vi "Ka2tesla - Hybrid.vi"(1 "SC Current [kA]":dbl format="%.5f", 2 "Current [KA]":dbl format="%.5f") -> (0 "Field":dbl=1.0 format="%.4f")   [LabVIEW 2020]
uses:
  PS Comm Globals.vi
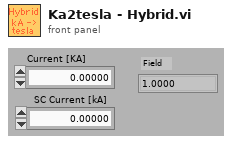
[diagram p1: front panel]
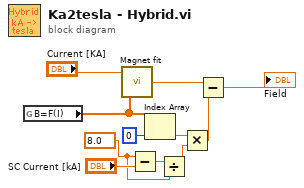
[diagram p0: block diagram]
diagram:
  w1 = 8.0 ("x")
  n1 = global read "PS Comm Globals.vi" "B=F(I)"() -> (w7:dbl[])
  n2 = call "Magnet fit.vi"("Coefficients"=w7, "Magnet Parameter"="Current [KA]") -> ("Conjugate Parameter"=w11:dbl)
  n3 = Subtract(x=w1, y="SC Current [kA]") -> (x-y=w2:dbl)
  n4 = Index Array(array=w7, index=0) -> (element=w6:dbl)
  n5 = Divide(x=w2, y=w1) -> (x/y=w3:dbl)
  n6 = Multiply(x=w6, y=w3) -> (x*y=w4:dbl)
  n7 = Subtract(x=w11, y=w4) -> (x-y=→"Field":dbl)
